vi "OpenByteStreamFileForReading.vi"(3 "File path to open":path) -> (0 "error out":errorcluster, 1 "Byte Stream File Refnum":refnum<file>)   [LabVIEW 2012]
panel:
  in  "open mode (0)":T1(ring)
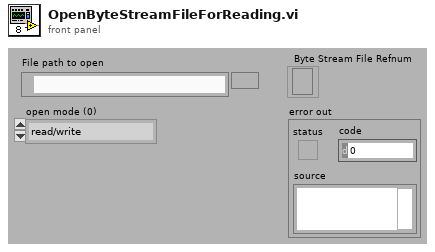
[diagram p1: front panel]
types:
  T1 = enum16{"read/write", "read-only", "write-only", "write-only (truncate)"}
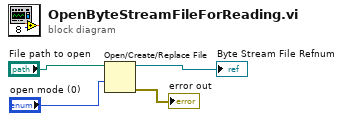
[diagram p0: block diagram]
diagram:
  n1 = Open/Create/Replace File(file path (use dialog)="File path to open", access (0:read/write)="open mode (0)") -> (refnum out=→"Byte Stream File Refnum":refnum<file>, error out=→"error out":errorcluster)  [unwired: 1 in, 4 out]
